vi "Open.vi"(8 "error in (no error)":errorcluster, 11 "Ini Path in":path) -> (0 "error out":errorcluster, 1 "Exists?":bool, 2 "skvc out":string[][](array[string]), 3 "Ini Path out":path)   [LabVIEW 2021, in "Config.lvlib"]
uses:
  Config.lvlib
  <vilib>/Utility/error.llb/Error Cluster From Error Code.vi
  <vilib>/ErrorRing/Error Ring.xnode
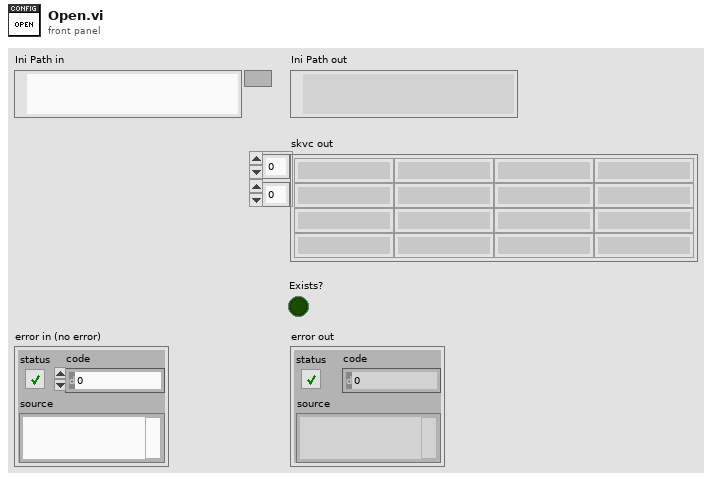
[diagram p1: front panel]
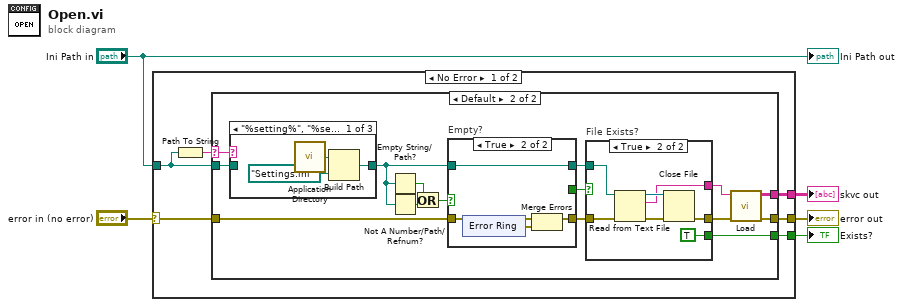
[diagram p0: block diagram]
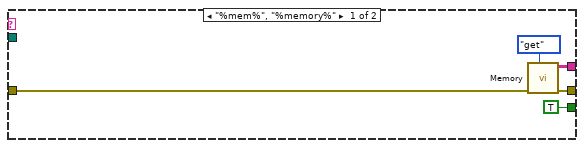
[diagram p2: hidden frame]
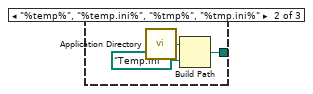
[diagram p3: hidden frame]
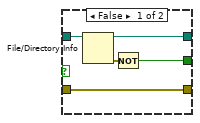
[diagram p6: hidden frame]
diagram:
  n1 = case shown="No Error" "error in (no error)" {
    selector: "error in (no error)" -> [w9 w60]
    tunnel: [w11 w60] -> w5
    tunnel: [w10 _] -> w4
    tunnel: "Ini Path in" -> [w7 _]
    tunnel: [w6 _] -> w1
    frame No Error {
      n2 = Path To String(path=w7) -> (string=w8:string)
      n3 = case shown="Default" w8 {
        selector: w8 -> [_ w17]
        tunnel: [w14 w31] -> w11
        tunnel: [w16 w30] -> w10
        tunnel: w9 -> [w13 w26]
        tunnel: w7 -> [_ w19]
        tunnel: [TRUE w20] -> w6
        frame "%mem%", "%memory%" {
          n4 = call "Memory.vi"("Action (get)"=enum8{"get", "set"}."get", "error in (no error)"=w13) -> ("error out"=w14:errorcluster, "skvc out"=w16:string[][])  [unwired: 8 in]
        }
        frame Default {
          n5 = case shown="\"%setting%\", \"%setting.ini%\", \"%settings%\", \"%settings.ini%\"" w17 {
            tunnel: w19 -> [_ _ w38]
            tunnel: [w34 w37 w38] -> w18
            frame "%setting%", "%setting.ini%", "%settings%", "%settings.ini%" {
              n6 = call <vilib>:"Application Directory.vi"() -> ("Application Directory"=w33:path)
              n7 = Build Path(base path=w33, name or relative path=path "Settings.ini") -> (appended path=w34:path)
            }
            frame "%temp%", "%temp.ini%", "%tmp%", "%tmp.ini%" {
              n8 = call <vilib>:"Application Directory.vi"() -> ("Application Directory"=w36:path)
              n9 = Build Path(base path=w36, name or relative path=path "Temp.ini") -> (appended path=w37:path)
            }
            frame Default {
            }
          }
          n10 = Empty String/Path?(string/path=w18) -> (empty?=w28:bool)
          n11 = Not A Number/Path/Refnum?(number/path/refnum=w18) -> (NaN/Path/Refnum?=w29:bool)
          n12 = Or(x=w28, y=w29) -> (x .or. y?=w27:bool)
          n13 = case "Empty?" shown="True" w27 {
            tunnel: w26 -> [w51 w55]
            tunnel: [w51 w54] -> w25
            tunnel: w18 -> [w50 w52]
            tunnel: [w48 w52] -> w23
            tunnel: [w47 _] -> w21
            frame False {
              n14 = File/Directory Info(path=w50) -> (path out=w48:path, error out=w49:errorcluster)  [unwired: 1 in, 5 out]
              n15 = Not(x=w49) -> (.not. x?=w47:bool)
            }
            frame True {
              n16 = xnode "Error Ring"() -> ("error out"=w53:errorcluster)
              n17 = Merge Errors(w55, w53) -> (w54:errorcluster)
            }
          }
          n18 = case "File Exists?" shown="True" w21 {
            tunnel: w25 -> [w39 w44]
            tunnel: [w39 w43] -> w24
            tunnel: w23 -> [_ w42]
            tunnel: [_ w41] -> w22
            tunnel: [_ TRUE] -> w20
            frame False {
            }
            frame True {
              n19 = Read from Text File(file (use dialog)=w42, error in=w44) -> (refnum out=w45:refnum<file>, text=w41:string, error out=w46:errorcluster)  [unwired: 2 in, 1 out]
              n20 = Close File(refnum=w45, error in=w46) -> (error out=w43:errorcluster)  [unwired: 1 out]
            }
          }
          n21 = call "Load.vi"("error in (no error)"=w24, "Text"=w22) -> ("error out"=w31:errorcluster, "skvc"=w30:string[][])  [unwired: 8 in]
        }
      }
    }
    frame Error {
    }
  }
  "error out" <- w5
  "skvc out" <- w4
  "Exists?" <- w1
  "Ini Path out" <- "Ini Path in"
